vi "UpdateTrendValueByID.vi"(9 "Value":dbl, 10 "TrendPoints id":string, 11 "TrendPoints in":T1[](array[typedef])) -> (3 "TrendPoints out":T1[](array[typedef]))   [LabVIEW 2017, in "McsaStartupAnalysis.lvlib"]
uses:
  <vilib>/addons/InsightCM/Devices/Shared/Mcsa/McsaStartupAnalysis/McsaStartupAnalysis.lvlib
  <vilib>/addons/InsightCM/MessageBus/Base/controls/TrendPoint.ctl
  <vilib>/addons/InsightCM/MessageBus/Base/controls/KeyValuePair.ctl
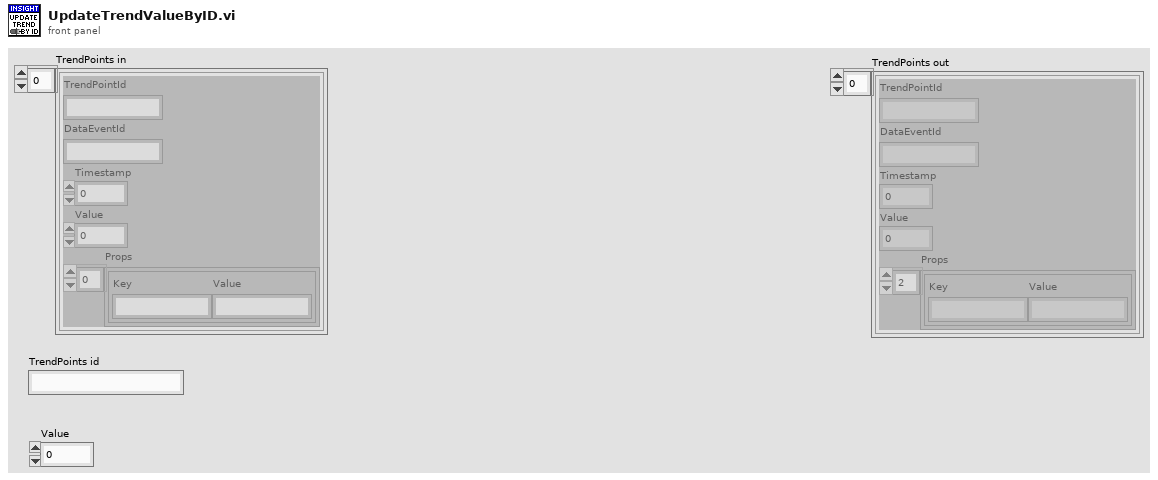
[diagram p1: front panel]
types:
  T1 = typedef "TrendPoint.ctl" = cluster{"TrendPointId":string, "DataEventId":string, "Timestamp":i64, "Value":dbl, "Props":T2[]}
  T2 = typedef "KeyValuePair.ctl" = cluster{"Key":string, "Value":string}
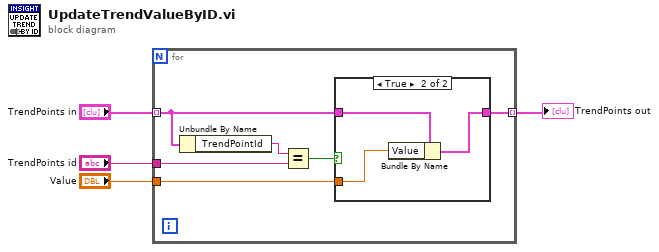
[diagram p0: block diagram]
diagram:
  n1 = for {
    tunnel: "TrendPoints in" -> [w8] mode=indexing
    tunnel: "TrendPoints id" -> [w9]
    tunnel: [w7] -> w1 mode=indexing
    tunnel: "Value" -> [w6]
    n2 = Unbundle By Name(w8) -> ("TrendPointId"=w10:string)
    n3 = Equal?(x=w10, y=w9) -> (x = y?=w5:bool)
    n4 = case shown="True" w5 {
      tunnel: w8 -> [w11 w14]
      tunnel: [w11 w13] -> w7
      tunnel: w6 -> [_ w12]
      frame False {
      }
      frame True {
        n5 = Bundle By Name(cluster=w14, "Value"=w12) -> (w13:T1)
      }
    }
  }
  "TrendPoints out" <- w1
